vi "displaying percentage using clusters.vi"() -> ()   [LabVIEW 2018]
panel:
  out "output cluster":T1
  in  "Cluster":T2
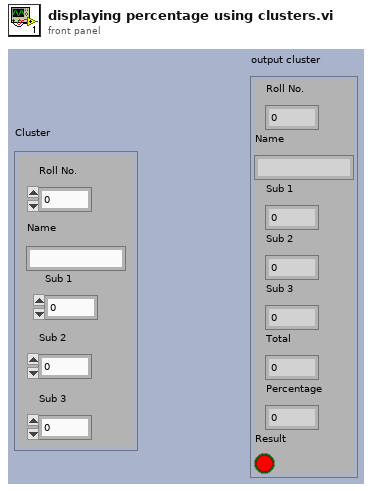
[diagram p1: front panel]
types:
  T1 = cluster{"Roll No.":i32, "Name":string, "Sub 1":i32, "Sub 2":i32, "Sub 3":i32, "Total":i32, "Percentage":dbl, "Result":bool}
  T2 = cluster{"Roll No.":u32, "Name":string, "Sub 1":u32, "Sub 2":u32, "Sub 3":u32}
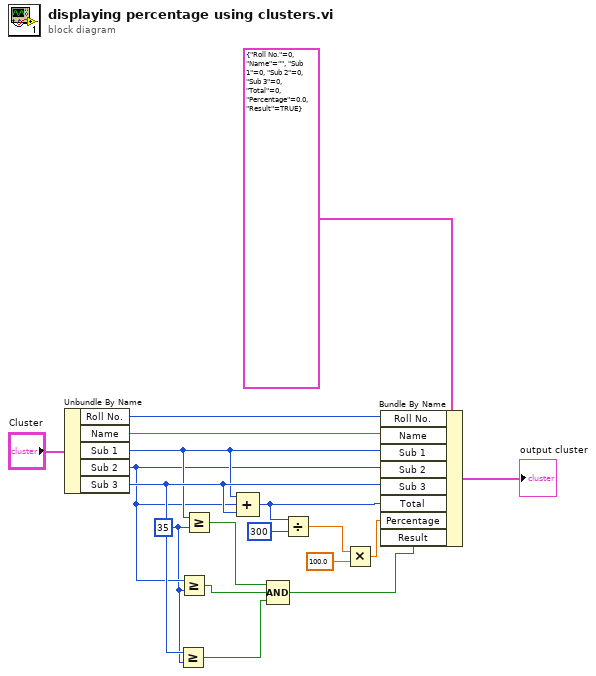
[diagram p0: block diagram]
diagram:
  w5 = u32 35 ("y")
  n1 = Unbundle By Name("Cluster") -> ("Roll No."=w18:u32, "Name"=w17:string, "Sub 1"=w7:u32, "Sub 2"=w6:u32, "Sub 3"=w8:u32)
  n2 = Greater Or Equal?(x=w8, y=w5) -> (x >= y?=w2:bool)
  n3 = Greater Or Equal?(x=w6, y=w5) -> (x >= y?=w3:bool)
  n4 = Greater Or Equal?(x=w7, y=w5) -> (x >= y?=w4:bool)
  n5 = Compound Arithmetic op=ADD(w7, w6, w8) -> (w12:u32)
  n6 = Compound Arithmetic op=AND(w4, w3, w2) -> (w1:bool)
  n7 = Divide(x=w12, y=u32 300) -> (x/y=w9:dbl)
  n8 = Multiply(x=w9, y=100.0) -> (x*y=w10:dbl)
  n9 = Bundle By Name(cluster=T1 {"Roll No."=0, "Name"="", "Sub 1"=0, "Sub 2"=0, "Sub 3"=0, "Total"=0, "Percentage"=0.0, "Result"=TRUE}, "Roll No."=w18, "Name"=w17, "Sub 1"=w7, "Sub 2"=w6, "Sub 3"=w8, "Total"=w12, "Percentage"=w10, "Result"=w1) -> (→"output cluster":T1)
